vi "Register Events to Controller.vi"(8 "error in (no error)":errorcluster, 11 "Example View in":refnum<class "Example View Actor.lvclass">) -> (0 "error out":errorcluster, 3 "Example View out":refnum<class "Example View Actor.lvclass">)   [LabVIEW 2016, in "Example View Actor.lvlib" / "Example View Actor.lvclass"]
doc: "This dinamic dispatch methods has to be overriddent by the child sink classes to register events to the source"
uses:
  Example View Actor.lvclass
  C:/Project/Shared Libraries/Event Actors/View Actor/View Actor.lvclass
  Example View Actor Messages/Update Array Event Msg/Update Array Event Msg.lvclass
  C:/Project/Shared Libraries/Event Actors/Event Handlers/Abstract Event Message for View/Abstract Event Message for View.lvclass
  Example Events/Double Array Event.lvclass
  C:/Project/Shared Libraries/Event Actors/Event/Event.lvclass
  Example View Actor Messages/Update Time Event Msg/Update Time Event Msg.lvclass
  Example Events/Timestamp Event.lvclass
  Example View Actor Messages/Update Boolean Event Msg/Update Boolean Event Msg.lvclass
  Example Events/Boolean Event.lvclass
  Event/Event.lvclass/Event.ctl
  View Actor/View Actor.lvclass/View Actor.ctl
  View Actor/properties/Read Controller Actor Enqueuer.vi
  View Actor/properties/Read Name.vi
  <vilib>/ActorFramework/Message Enqueuer/Message Enqueuer.lvclass
  Event/Event.lvclass
  Controller Actor Messages/Register by Name Msg/Register by Name Msg.lvclass
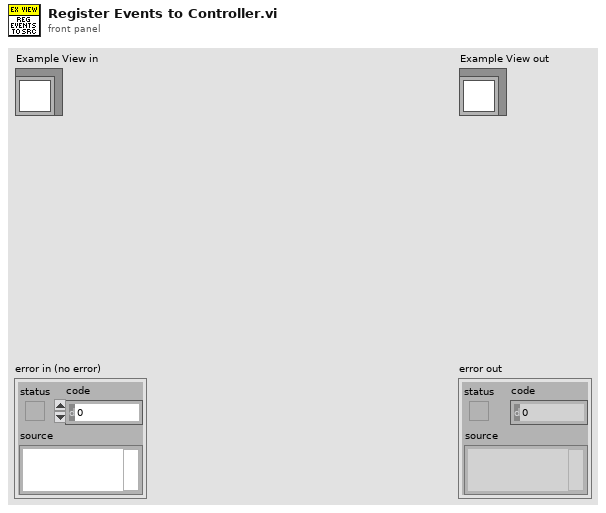
[diagram p1: front panel]
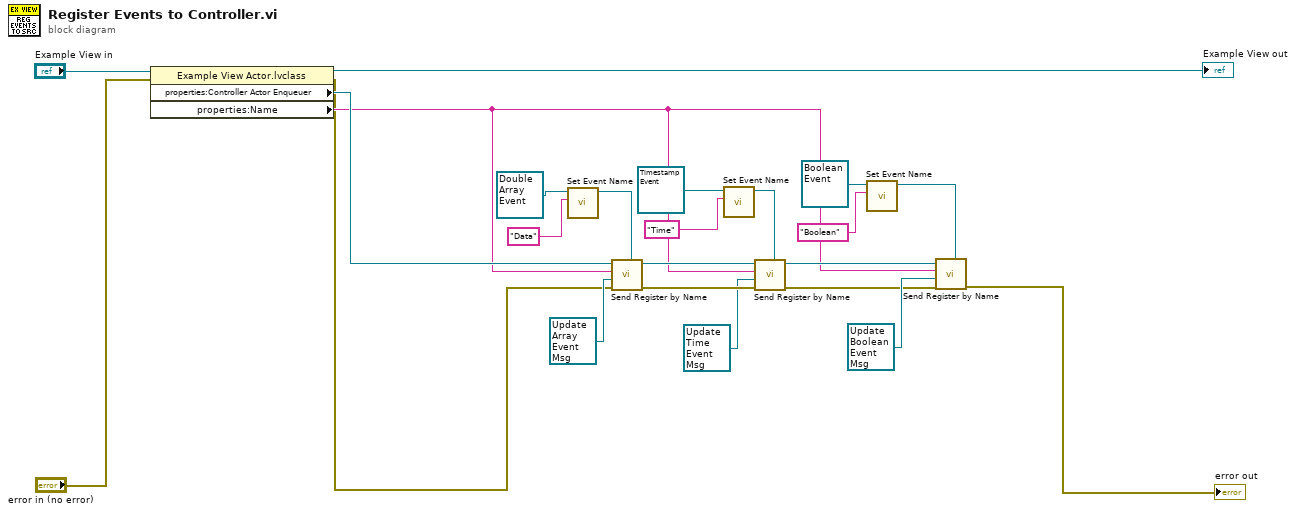
[diagram p0: block diagram]
diagram:
  n1 = property class="Example View Actor.lvclass"(reference="Example View in", error in="error in (no error)") -> (reference out=→"Example View out":refnum<class "Example View Actor.lvclass">, error out=w5:errorcluster, "properties:Controller Actor Enqueuer"=w7:refnum<class "Message Enqueuer.lvclass">, "properties:Name"=w6:string)
  n2 = call "Set Event Name.vi"("Name (Generic)"="Data", "Event In"=refnum<class "Double Array Event.lvclass"> refnum ("Double Array Event.lvclass")) -> ("Event Out"=w17:refnum<class "Double Array Event.lvclass">)  [unwired: 9 in]
  n3 = call "Send Register by Name.vi"("Event"=w17, "error in (no error)"=w5, "Event Fire Handler"=refnum<class "Update Array Event Msg.lvclass"> refnum ("Update Array Msg.lvclass"), "View Name"=w6, "Message Enqueuer in"=w7) -> ("error out"=w11:errorcluster, "Message Enqueuer out"=w13:refnum<class "Message Enqueuer.lvclass">)  [unwired: 5 in]
  n4 = call "Set Event Name.vi"("Name (Generic)"="Time", "Event In"=refnum<class "Timestamp Event.lvclass"> refnum ("Timestamp Event.lvclass")) -> ("Event Out"=w8:refnum<class "Timestamp Event.lvclass">)  [unwired: 9 in]
  n5 = call "Send Register by Name.vi"("Event"=w8, "error in (no error)"=w11, "Event Fire Handler"=refnum<class "Update Time Event Msg.lvclass"> refnum ("Update Time Msg.lvclass"), "View Name"=w6, "Message Enqueuer in"=w13) -> ("error out"=w10:errorcluster, "Message Enqueuer out"=w12:refnum<class "Message Enqueuer.lvclass">)  [unwired: 5 in]
  n6 = call "Set Event Name.vi"("Name (Generic)"="Boolean", "Event In"=refnum<class "Boolean Event.lvclass"> refnum ("Example Source.lvlib:Boolean Event.lvclass")) -> ("Event Out"=w15:refnum<class "Boolean Event.lvclass">)  [unwired: 9 in]
  n7 = call "Send Register by Name.vi"("Event"=w15, "error in (no error)"=w10, "Event Fire Handler"=refnum<class "Update Boolean Event Msg.lvclass"> refnum ("Update Time Msg.lvclass"), "View Name"=w6, "Message Enqueuer in"=w12) -> ("error out"=→"error out":errorcluster)  [unwired: 5 in, 1 out]
